vi "Update Values.vi"(6 "Timestamp (Now)":dbl, 8 "error in (no error)":errorcluster, 9 "Raw Values (N/A)":dbl[](array[numeric]), 10 "Values":dbl[](array[numeric]), 11 "Group in":refnum<class "Group.lvclass">) -> (0 "error out":errorcluster, 3 "Group out":refnum<class "Group.lvclass">)   [LabVIEW 2020, in "Vecto.lvlib" / "Group.lvclass"]
uses:
  Group.lvclass
  Group.lvclass/Group.ctl
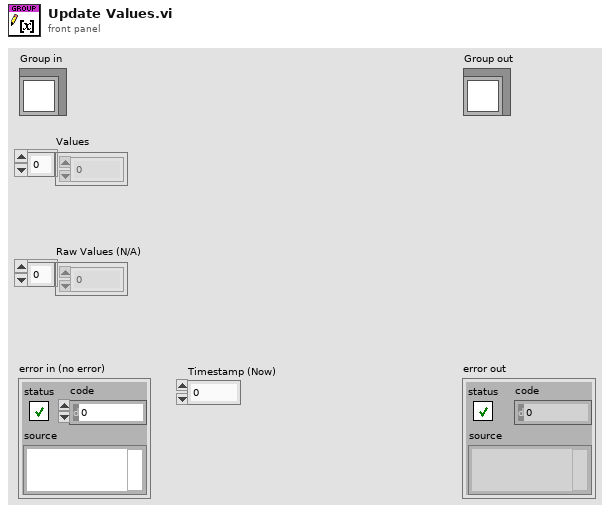
[diagram p1: front panel]
types:
  T1 = typedef "Vecto.lvlib/Group.lvclass/Ref.ctl" = cluster{"Channels":refnum<data-value>[], "Channel Index Map":map{string, i32}}
  T2 = typedef "Vecto.lvlib/Channel.ctl" = cluster{"Info":T3, "Value":T4}
  T3 = typedef "Vecto.lvlib/Channel Info.ctl" = cluster{"Name":string, "Group":string, "Owning Node":u32, "Owning Task":u32, "Resource":string}
  T4 = typedef "Vecto.lvlib/Channel Value.ctl" = cluster{"Scaled":dbl, "Timestamp":dbl, "Raw":dbl}
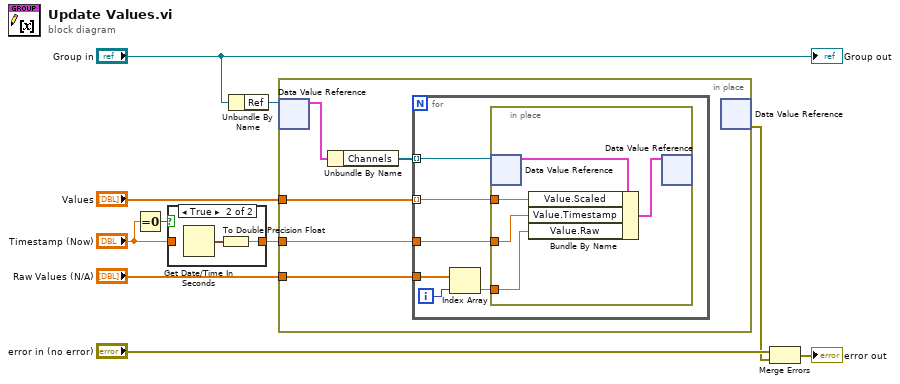
[diagram p0: block diagram]
diagram:
  n1 = Equal To 0?(x="Timestamp (Now)") -> (x = 0?=w5:bool)
  n2 = case shown="True" w5 {
    tunnel: "Timestamp (Now)" -> [w11 _]
    tunnel: [w11 w12] -> w3
    frame False {
    }
    frame True {
      n3 = Get Date/Time In Seconds() -> (seconds since 1Jan1904=w13:timestamp)
      n4 = To Double Precision Float(number=w13) -> (double precision float=w12:dbl)
    }
  }
  n5 = Unbundle By Name("Group in") -> ("Ref"=w8:refnum<data-value>)
  n6 = in-place {
    in-place-border: "Values" -> [w16]
    in-place-border: "Raw Values (N/A)" -> [w14]
    in-place-border: w3 -> [w15]
    n7 = in-place-dvr #1(w8) -> (w18:T1)  [unwired: 1 out]
    n8 = Unbundle By Name(w18) -> ("Channels"=w17:refnum<data-value>[])
    n9 = for {
      tunnel: w17 -> [w24] mode=indexing
      tunnel: w16 -> [w23] mode=indexing
      tunnel: w15 -> [w22]
      tunnel: w14 -> [w21]
      i -> [w20]
      n10 = Index Array(array=w21, index=w20) -> (element=w19:dbl)
      n11 = in-place {
        in-place-border: w23 -> [w28]
        in-place-border: w22 -> [w27]
        in-place-border: w19 -> [w26]
        n12 = in-place-dvr #2(w24) -> (w29:T2)  [unwired: 1 out]
        n13 = Bundle By Name(cluster=w29, "Value.Scaled"=w28, "Value.Timestamp"=w27, "Value.Raw"=w26) -> (w25:T2)
        n14 = in-place-dvr #2(w25) -> ()  [unwired: 2 out]
      }
    }
    n15 = in-place-dvr #1() -> (w1:errorcluster)  [unwired: 1 in, 1 out]
  }
  n16 = Merge Errors("error in (no error)", w1) -> (→"error out":errorcluster)
  "Group out" <- "Group in"
